vi "AllShareVariable.vi"() -> ()   [LabVIEW 2010]
uses:
  Ctrls/ServerData.ctl
  Ctrls/DeviceInfomation.ctl
  Ctrls/DeviceModel.ctl
  Ctrls/ChannelData.ctl
  Ctrls/ChannelType.ctl
  Ctrls/ChannelAccessType.ctl
  SubVIs/ModBUS Driver/Private/MBDRV_Response List.ctl
  SubVIs/ModBUS Driver/Private/MBDRV_Response.ctl
  SubVIs/ModBUS Driver/Private/MBDRV_Action.ctl
  SubVIs/ModBUS Driver/Private/MBDRV_Command List.ctl
  SubVIs/ModBUS Driver/Private/MBDRV_Command Data.ctl
  Drivers/ModbusServer/DeviceListChannelData.ctl
  Drivers/ModbusServer/AutoChannelData.ctl
  Drivers/ModbusServer/DeviceListModbusAddressRegister.ctl
  Drivers/ModbusServer/ModbusAddressRegister.ctl
  Drivers/ModbusServer/MonitorServer.lvlib
panel:
  out "DeviceListRegister":T1
  out "AutoReadChannels":T3
  in  "Write To PLC":T5
  out "Read From PLC":T8
  in  "Server Status":string
  in  "ServerData":T10
  in  "CurrentDeviceName":string
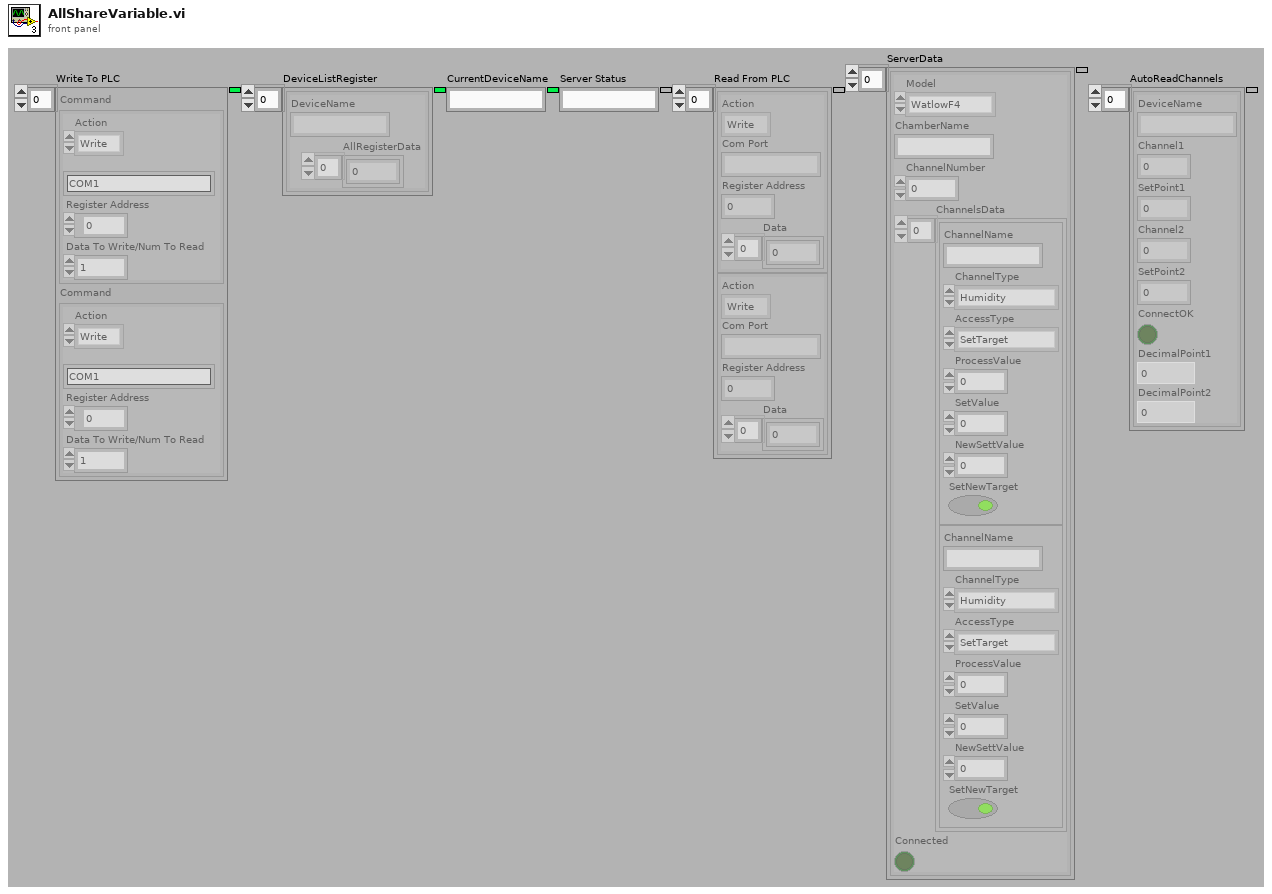
[diagram p1: front panel]
types:
  T1 = typedef "MonitorServer.lvlib/DeviceListModbusAddressRegister.ctl" = T2[]
  T2 = typedef "MonitorServer.lvlib/ModbusAddressRegister.ctl" = cluster{"DeviceName":string, "AllRegisterData":i16[]}
  T3 = typedef "MonitorServer.lvlib/DeviceListChannelData.ctl" = T4[]
  T4 = typedef "MonitorServer.lvlib/AutoChannelData.ctl" = cluster{"DeviceName":string, "Channel1":dbl, "SetPoint1":dbl, "Channel2":dbl, "SetPoint2":dbl, "ConnectOK":bool, "DecimalPoint1":i16, "DecimalPoint2":i16}
  T5 = typedef "MBDRV_Command List.ctl" = T6[]
  T6 = typedef "MBDRV_Command Data.ctl" = cluster{"Action":T7, "Com Port":string, "Register Address":u16, "Data To Write/Num To Read":i16}
  T7 = typedef "MBDRV_Action.ctl" = enum16{"Write", "Read"}
  T8 = typedef "MBDRV_Response List.ctl" = T9[]
  T9 = typedef "MBDRV_Response.ctl" = cluster{"Action":T7, "Com Port":string, "Register Address":u16, "Data":i16[]}
  T10 = typedef "ServerData.ctl" = T11[]
  T11 = typedef "DeviceInfomation.ctl" = cluster{"Model":T12, "ChamberName":string, "ChannelNumber":i32, "ChannelsData":T13[], "Connected":bool}
  T12 = typedef "DeviceModel.ctl" = enum16{"WatlowF4", "CenterOne", "DCP551", "DPR250"}
  T13 = typedef "ChannelData.ctl" = cluster{"ChannelName":string, "ChannelType":T14, "AccessType":T15, "ProcessValue":dbl, "SetValue":dbl, "NewSettValue":dbl, "SetNewTarget":bool}
  T14 = typedef "ChannelType.ctl" = enum16{"Temperature", "Humidity"}
  T15 = typedef "ChannelAccessType.ctl" = enum16{"ReadOnly", "SetTarget"}
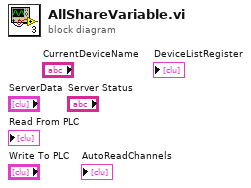
[diagram p0: block diagram]
diagram:
